vi "Inv Chi Square Distribution.vi"(2 "degrees of freedom":i32=1 format="%0.0f", 3 "probability":dbl format="%0.4f") -> (0 "error":i32, 1 "x":dbl format="%0.4f")   [LabVIEW 2017, in "NI_AALPro.lvlib"]
doc: "LabVIEW no longer supports this VI. Use the Continuous Inverse CDF VI (Chi-Squared instance) instead. Computes the value of <B>x</B> given the <B>probability</B> value, p, of a chi-square-distributed random variable, X, with n <B>degrees of freedom</B>. The Inv Chi Square Distribution VI computes the value of <B>x</B> such that the following condition is satisfied: p = Prob{X <= <B>x</B>}, where X is Chi squared distributed with n <B>degrees of freedom</B>, p is the <B>probability</B>, and <B>x</B> is the value."
uses:
  <vilib>/Analysis/NI_AALPro.lvlib
  <resource>/lvanlys.dll
panel:
  # "Inverse Chi-Square\nDistribution"
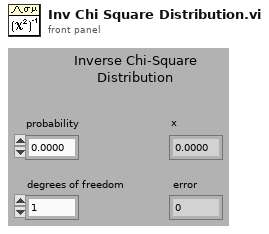
[diagram p1: front panel]
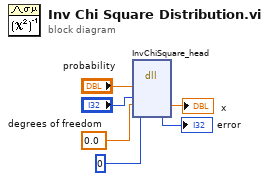
[diagram p0: block diagram]
diagram:
  n1 = dll-call lib="e:/builds/penguin/labview/branches/2017/dev/dist/resource/lvanlys.*" fn="InvChiSquare_head"("probability"="probability", "degrees of freedom"="degrees of freedom", 0.0, 0) -> (→"x":dbl, →"error":i32)  [unwired: 6 in, 2 out]
